vi "Force_reference_R.vi"(0 "Initialize":bool, 1 "Force_peak":sgl, 5 "FPGA_data":sgl[](array[numeric])=[0.0, 0.0, 0.0, 0.0, 0.0, 0.0, 0.0, 0.0, 0.0, 0.0, 0.0, 0.0, 0.0, 0.0, 0.0, 0.0, 0.0, 0.0, 0.0, 0.0, 0.0, 0.0, 0.0, 0.0, 0.0, 0.0, 0.0, 0.0, 0.0, 0.0, 0.0], 7 "출력 클러스터 2":T1, 9 "R_power_raw":sgl, 11 "에러 입력":errorcluster caption="에러 출력") -> (2 "CAN":enum16{"stand", "init", "read"}(ring), 3 "R_power_OK":bool, 4 "Force_ref_R":sgl, 8 "출력 클러스터":T1, 15 "에러 출력":errorcluster)   [LabVIEW 2019]
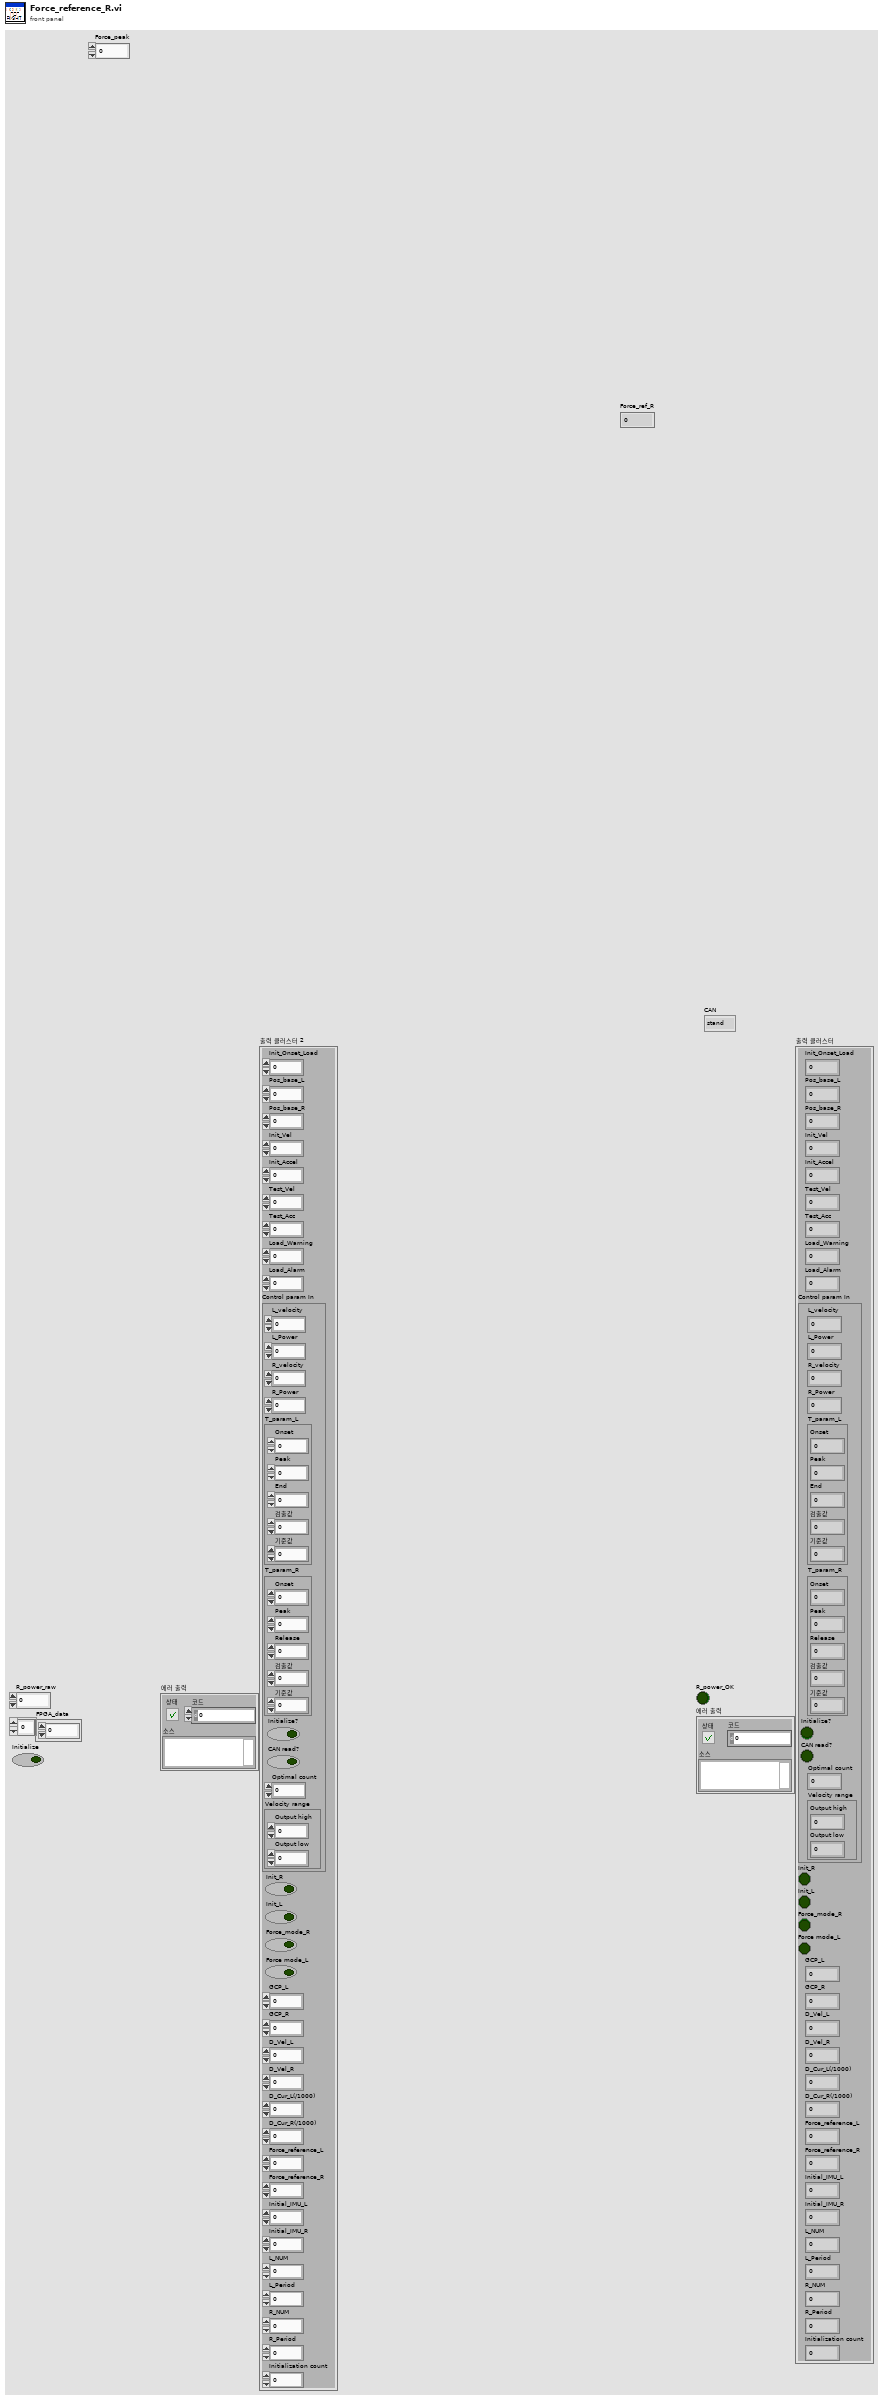
[diagram p1: front panel]
types:
  T1 = cluster{"Init_Onset_Load":sgl, "Pos_base_L":sgl, "Pos_base_R":sgl, "Init_Vel":i32, "Init_Accel":u32, "Test_Vel":i32, "Test_Acc":u32, "Load_Warning":sgl, "Load_Alarm":sgl, "Control param In":cluster{"L_velocity":u32, "L_Power":sgl, "R_velocity":u32, "R_Power":sgl, "T_param_L":cluster{"Onset":sgl, "Peak":sgl, "End":sgl, "검출값":sgl, "기준값":sgl}, "T_param_R":cluster{"Onset":sgl, "Peak":sgl, "Release":sgl, "검출값":sgl, "기준값":sgl}, "Initialize?":bool, "CAN read?":bool, "Optimal count":i32, "Velocity range":cluster{"Output high":dbl, "Output low":dbl}}, "Init_R":bool, "Init_L":bool, "Force_mode_R":bool, "Force mode_L":bool, "GCP_L":sgl, "GCP_R":sgl, "D_Vel_L":sgl, "D_Vel_R":sgl, "D_Cur_L(/1000)":sgl, "D_Cur_R(/1000)":sgl, "Force_reference_L":sgl, "Force_reference_R":sgl, "Initial_IMU_L":sgl, "Initial_IMU_R":sgl, "L_NUM":u32, "L_Period":i16, "R_NUM":u32, "R_Period":i16, "Initialization count":i32}
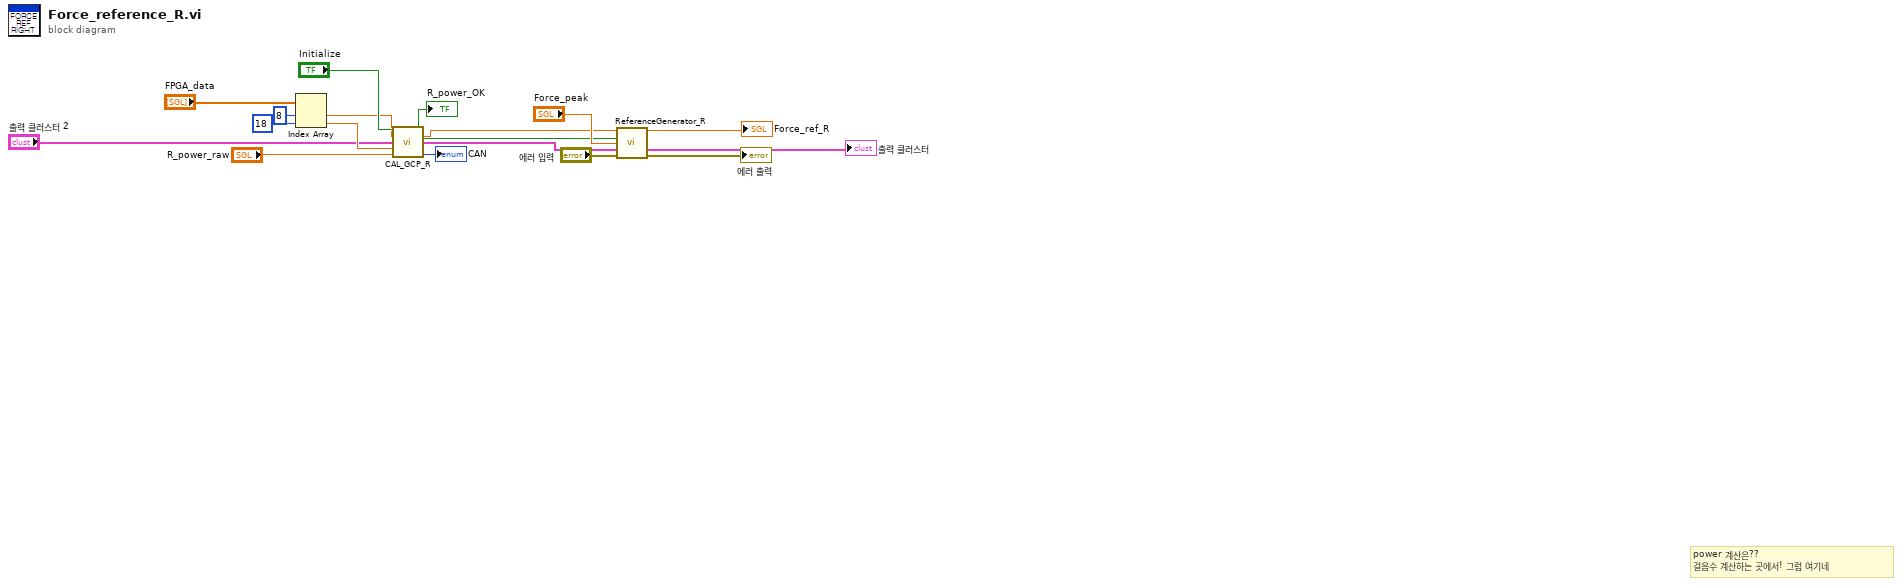
[diagram p0: block diagram]
diagram:
  # "power 계산은??\n걸음수 계산하는 곳에서! 그럼 여기네"
  n1 = Index Array(array="FPGA_data", index #1=8 ("인덱스"), index #2=18 ("인덱스")) -> (element #1=w14:sgl, element #2=w13:sgl)
  n2 = call "CAL_GCP_R.vi"("Initialize"="Initialize", "R_ROLL"=w14, "출력 클러스터 2"="출력 클러스터 2", "B_ACC"=w13, "R_power_raw"="R_power_raw") -> ("R_power_OK"=→"R_power_OK":bool, "R_Ctrl_Start"=w4:bool, "R_GCP"=w3:sgl, "출력 클러스터"=w5:T1, "CAN"=→"CAN":enum16{"stand", "init", "read"})  [unwired: 5 in, 1 out]
  n3 = call "ReferenceGenerator_R.vi"("GCP_1k_R"=w3, "R_ctl_start"=w4, "Force_peak"="Force_peak", "출력 클러스터 2"=w5, "에러 출력"="에러 입력") -> ("Force_ref_R"=→"Force_ref_R":sgl, "출력 클러스터"=→"출력 클러스터":T1, "에러 출력 2"=→"에러 출력":errorcluster)  [unwired: 8 in]
